vi "Write Path.vi"(8 "error in (no error)":errorcluster, 10 "Path":path, 11 "bin datalogger configuration in":refnum<class "Binary datalogger configuration.lvclass">) -> (0 "error out":errorcluster, 3 "bin datalogger configuration out":refnum<class "Binary datalogger configuration.lvclass">)   [LabVIEW 2013, in "Binary datalogger configuration.lvclass"]
uses:
  Binary datalogger configuration.lvclass
  Binary datalogger configuration.lvclass/Binary datalogger configuration.ctl
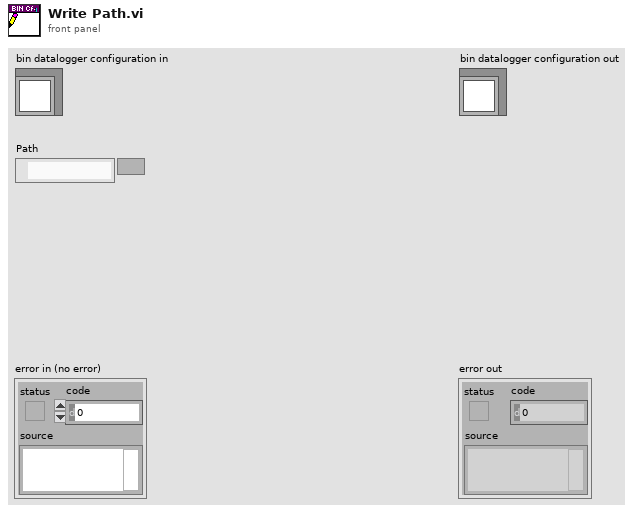
[diagram p1: front panel]
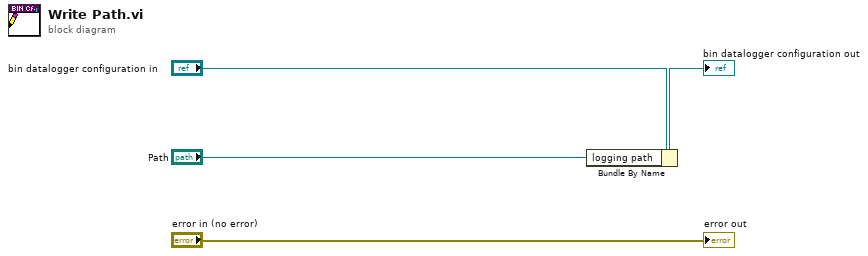
[diagram p0: block diagram]
diagram:
  n1 = Bundle By Name(cluster="bin datalogger configuration in", "logging path"="Path") -> (→"bin datalogger configuration out":refnum<class "Binary datalogger configuration.lvclass">)
  "error out" <- "error in (no error)"
